vi "Periodic Random Noise.vi"(2 "seed":i32=-1, 3 "spectral amplitude":dbl=1.0 format="%0.2f", 4 "samples":i32=128) -> (0 "error":i32, 1 "periodic random noise":dbl[](array[numeric]))   [LabVIEW 2014, in "NI_AALBase.lvlib"]
doc: "Generates an array containing periodic random noise (PRN)."
uses:
  NI_AALBase.lvlib
  lvanlys.dll
panel:
  # "Periodic Random Noise"
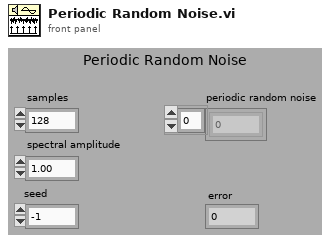
[diagram p1: front panel]
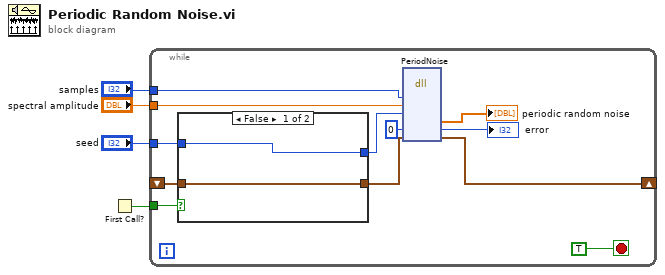
[diagram p0: block diagram]
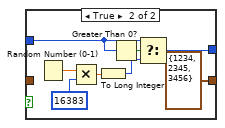
[diagram p2: hidden frame]
diagram:
  n1 = First Call?() -> (First Call?: T/F=w4:bool)
  n2 = while {
    shift-right: [w7] -> _
    shift-left: _ -> [w10]
    tunnel: w4 -> [w9]
    tunnel: "spectral amplitude" -> [w14]
    tunnel: "samples" -> [w13]
    tunnel: "seed" -> [w12]
    stop <- TRUE stop-if-true
    n3 = case shown="False" w9 {
      tunnel: w10 -> [w18 _]
      tunnel: [w18 cluster{"xSeed":i32, "ySeed":i32, "zSeed":i32} {"xSeed"=1234, "ySeed"=2345, "zSeed"=3456} ("RNGState")] -> w8
      tunnel: [w17 w24] -> w11
      tunnel: w12 -> [w17 w25]
      frame False {
      }
      frame True {
        n4 = Random Number (0-1)() -> (number: 0 to 1=w22:dbl)
        n5 = Multiply(x=w22, y=16383 ("x")) -> (x*y=w23:dbl)
        n6 = To Long Integer(number=w23) -> (32bit integer=w21:i32)
        n7 = Greater Than 0?(x=w25) -> (x > 0?=w26:bool)
        n8 = Select(t=w25, s=w26, f=w21) -> (s? t:f=w24:i32)
      }
    }
    n9 = dll-call lib="C:/Program Files (x86)/National Instruments/LabVIEW 2014/resource/lvanlys.*" fn="PeriodNoise"("samples"=w13, "spectral amplitude"=w14, "seed"=w11, "error"=0, "RNGState"=w8) -> ("periodic random noise"=→"periodic random noise":dbl[], "error"=→"error":i32, "RNGState"=w7:cluster{"xSeed":i32, "ySeed":i32, "zSeed":i32})  [unwired: 8 in, 2 out]
  }
